vi "onLeave.vi"(8 "error in (no error)":errorcluster, 11 "Filled Text Fields Actor in":refnum<class "Filled Text Fields Actor.lvclass">) -> (0 "error out":errorcluster, 3 "Filled Text Fields Actor out":refnum<class "Filled Text Fields Actor.lvclass">)   [LabVIEW 2017, in "Filled Text Fields.lvlib" / "Filled Text Fields Actor.lvclass"]
uses:
  Filled Text Fields Actor.lvclass
  Filled Text Fields.States.ctl
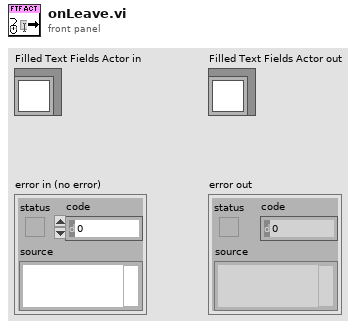
[diagram p1: front panel]
types:
  T1 = typedef "Filled Text Fields.lvlib/Filled Text Fields Actor.lvclass/Filled Text Fields.States.ctl" = enum16{"Inactive", "Activated", "Error", "Focused", "Hover", "Disabled", "Disabled and Grey out"}
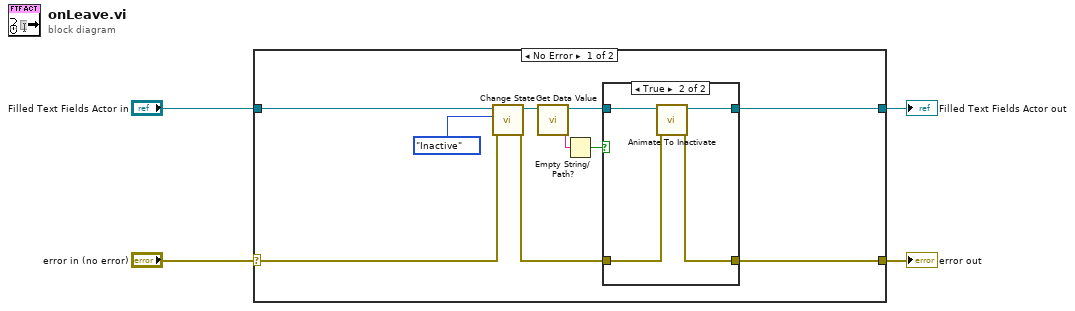
[diagram p0: block diagram]
diagram:
  n1 = case shown="No Error" "error in (no error)" {
    selector: "error in (no error)" -> [w13 w22]
    tunnel: [w9 w22] -> w3
    tunnel: [w11 w21] -> w1
    tunnel: "Filled Text Fields Actor in" -> [w14 w21]
    frame No Error {
      n2 = call "Change State.vi"("error in (no error)"=w13, "New State"=Filled_Text_Fields.States."Inactive", "Filled Text Fields Actor in"=w14) -> ("error out"=w10:errorcluster, "Filled Text Fields Actor out"=w12:refnum<class "Filled Text Fields Actor.lvclass">)  [unwired: 7 in]
      n3 = call "Get Data Value.vi"("Filled Text Fields Actor in"=w12) -> ("Value"=w6:string, "Filled Text Fields Actor out"=w7:refnum<class "Filled Text Fields Actor.lvclass">)  [unwired: 9 in]
      n4 = Empty String/Path?(string/path=w6) -> (empty?=w5:bool)
      n5 = case shown="True" w5 {
        tunnel: [w16 w20] -> w11
        tunnel: w10 -> [w15 w19]
        tunnel: [w15 w18] -> w9
        tunnel: w7 -> [w16 w17]
        frame False {
        }
        frame True {
          n6 = call "Animate To Inactivate.vi"("error in (no error)"=w19, "Filled Text Fields Actor in"=w17) -> ("error out"=w18:errorcluster, "Filled Text Fields Actor out"=w20:refnum<class "Filled Text Fields Actor.lvclass">)  [unwired: 8 in]
        }
      }
    }
    frame Error {
    }
  }
  "error out" <- w3
  "Filled Text Fields Actor out" <- w1
